vi "Destroy.vi"(8 "error in (no error)":errorcluster, 11 "CS++Reference in":refnum<class "CS++Reference.lvclass">) -> (0 "error out":errorcluster, 2 "Valid?":bool, 3 "Object":refnum<class "CS++Base.lvclass">)   [LabVIEW 2012, in "CS++BaseClasses.lvlib" / "CS++Reference.lvclass"]
doc: "Destroy queue and return contained object."
uses:
  CS++Reference.lvclass
  Base/CS++Base.lvclass
  CS++Reference.lvclass/CS++Reference.ctl
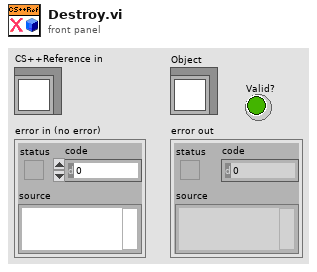
[diagram p1: front panel]
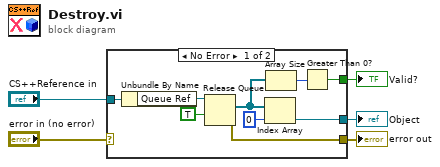
[diagram p0: block diagram]
diagram:
  n1 = case shown="No Error" "error in (no error)" {
    selector: "error in (no error)" -> [_ w15]
    tunnel: [w11 w15] -> w4
    tunnel: [w9 _] -> w2
    tunnel: "CS++Reference in" -> [w14 _]
    tunnel: [w6 _] -> w1
    frame No Error {
      n2 = Unbundle By Name(w14) -> ("Queue Ref"=w13:refnum<queue>)
      n3 = Release Queue(queue=w13, force destroy? (F)=TRUE) -> (remaining elements=w8:refnum<class "CS++Base.lvclass">[], error out=w11:errorcluster)  [unwired: 1 in, 1 out]
      n4 = Index Array(array=w8, index=0) -> (element=w9:refnum<class "CS++Base.lvclass">)
      n5 = Array Size(array=w8) -> (size(s)=w7:i32)
      n6 = Greater Than 0?(x=w7) -> (x > 0?=w6:bool)
    }
    frame Error {
    }
  }
  "error out" <- w4
  "Object" <- w2
  "Valid?" <- w1
